vi "DB FGV.vi"() -> (3 "DB ref":T1)   [LabVIEW 2024]
uses:
  <vilib>/addons/database/Connection.llb/Conn ObjectReference.ctl
  CTRLS/DB operation Selector.ctl
  CTRLS/GLB_VAR.vi
  <vilib>/addons/database/Connection.llb/DB Tools Open Connec (String).vi
  <vilib>/addons/database/NI_Database_API.lvlib
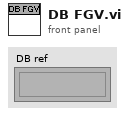
[diagram p1: front panel]
types:
  T1 = typedef "NI_Database_API.lvlib/Conn ObjectReference.ctl" = refnum<k1>
  T2 = typedef "DB operation Selector.ctl" = enum16{"Select", "Insert", "Update", "Execute select Query", "Execute update query"}
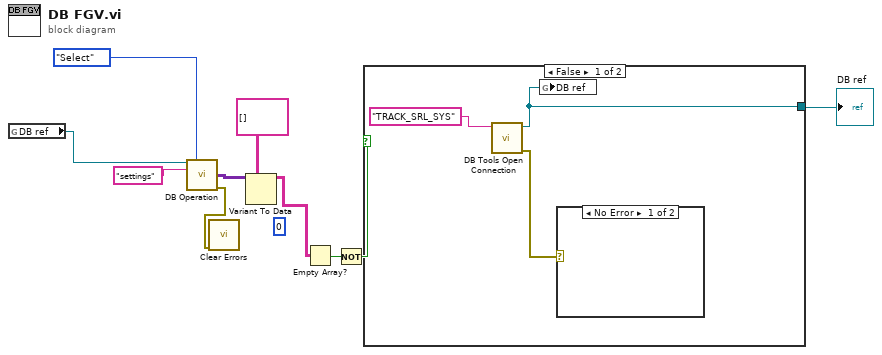
[diagram p0: block diagram]
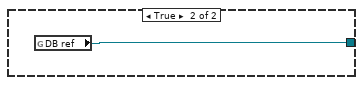
[diagram p3: hidden frame]
diagram:
  (unwired) 0 ("index (col)")
  n1 = global read "GLB_VAR.vi" "DB ref"() -> (w8:T1)
  n2 = call "DB Operation.vi"("connection reference"=w8, "DB Op Selector"=DB_operation_Selector."Select", "table"="settings") -> ("data out"=w5:variant[][], "error out"=w1:errorcluster)  [unwired: 10 in, 1 out]
  n3 = call <vilib>:"Clear Errors.vi"("error in (no error)"=w1) -> ()  [unwired: 5 in, 2 out]
  n4 = Variant To Data(type=string[][] [], Variant=w5) -> (data=w4:string[][])  [unwired: 1 in, 1 out]
  n5 = Empty Array?(array=w4) -> (empty?=w3:bool)
  n6 = Not(x=w3) -> (.not. x?=w2:bool)
  n7 = case shown="False" w2 {
    tunnel: [w12 w14] -> w10
    frame False {
      n8 = call-poly <vilib>:"DB Tools Open Connection.vi"("connection information"="TRACK_SRL_SYS" ("table")) -> ("error out"=w13:errorcluster, "connection reference"=w12:T1)  [unwired: 7 in]
      n9 = global write "GLB_VAR.vi" "DB ref"(w12) -> ()
      n10 = case shown="No Error" w13 {
        frame No Error {
        }
        frame Error {
        }
      }
    }
    frame True {
      n11 = global read "GLB_VAR.vi" "DB ref"() -> (w14:T1)
    }
  }
  "DB ref" <- w10
